vi "haveOneStart.vi"(2 "Byte Array":u8[](array[numeric]), 3 "Length":i32) -> (0 "offset":i32, 1 "match substring":string)   [LabVIEW 2014]
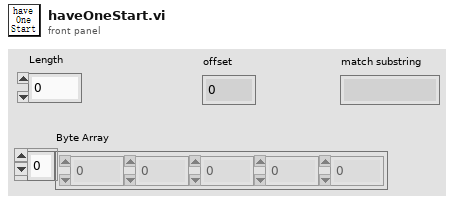
[diagram p1: front panel]
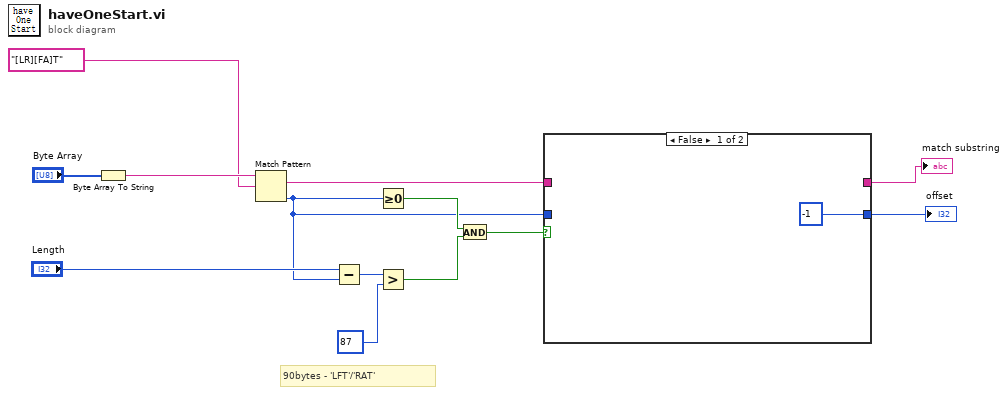
[diagram p0: block diagram]
diagram:
  # "90bytes - 'LFT'/'RAT'"
  n1 = Byte Array To String(unsigned byte array="Byte Array") -> (string=w13:string)
  n2 = Match Pattern(string=w13, regular expression="[LR][FA]T") -> (match substring=w1:string, offset past match=w4:i32)  [unwired: 1 in, 2 out]
  n3 = Subtract(x="Length", y=w4) -> (x-y=w10:i32)
  n4 = Greater Or Equal To 0?(x=w4) -> (x >= 0?=w9:bool)
  n5 = Greater?(x=w10, y=87) -> (0:w8:bool)
  n6 = And(x=w9, y=w8) -> (x .and. y?=w6:bool)
  n7 = case shown="False" w6 {
    tunnel: [-1 w16] -> w5
    tunnel: w4 -> [_ w16]
    tunnel: [_ w15] -> w2
    tunnel: w1 -> [_ w15]
    frame False {
    }
    frame True {
    }
  }
  "offset" <- w5
  "match substring" <- w2
